vi "Write S8.vi"(0 "I2C In":refnum<class "I2C.lvclass">, 1 "Slave Address":u8, 5 "Register":u32, 9 "Value":i8, 11 "Error In":errorcluster, 12 "Register Size":T1) -> (4 "I2C Out":refnum<class "I2C.lvclass">, 15 "Error Out":errorcluster)   [LabVIEW 2020, in "lv_i2c_hal.lvlib" / "I2C.lvclass"]
uses:
  I2C.lvclass
  Register Address Size.ctl
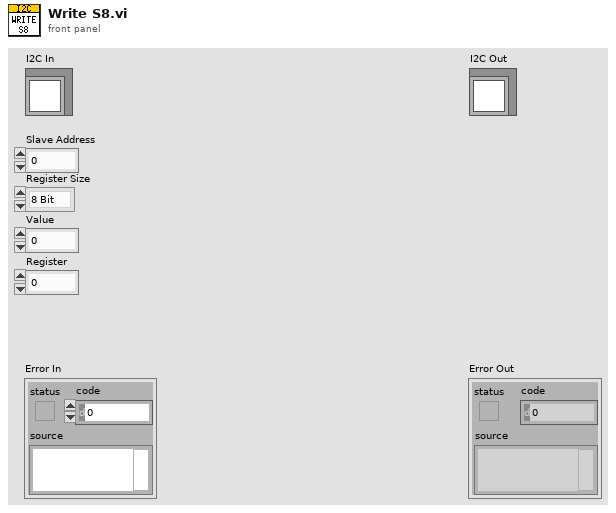
[diagram p1: front panel]
types:
  T1 = typedef "lv_i2c_hal.lvlib/I2C.lvclass/Register Address Size.ctl" = enum16{"8 Bit", "16 Bit", "24 Bit", "32 Bit"}
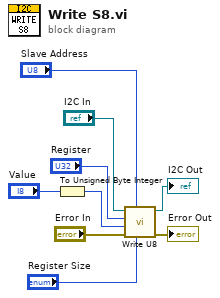
[diagram p0: block diagram]
diagram:
  n1 = To Unsigned Byte Integer(number="Value") -> (unsigned 8bit integer=w1:u8)
  n2 = call "Write U8.vi"("Register Size"="Register Size", "Slave Address"="Slave Address", "Error In"="Error In", "Value"=w1, "Register"="Register", "I2C In"="I2C In") -> ("Error Out"=→"Error Out":errorcluster, "I2C Out"=→"I2C Out":refnum<class "I2C.lvclass">)  [unwired: 4 in]
